vi "Render Inverted Section with Null.vi"(8 "Error In":errorcluster) -> (0 "Error Out":errorcluster)   [LabVIEW 2018, in "Tests.lvlib" / "Render.lvlib"]
uses:
  Render.lvlib
  <vilib>/addons/_JKI Toolkits/Caraya/classes/Test/Test.lvclass
  <vilib>/addons/_JKI Toolkits/Caraya/classes/Assert/Assert.lvclass
  src/Toolkit/Toolkit.lvlib
  src/Toolkit/Low-Level/Support/Render to String.vi
  src/Toolkit/Low-Level/Support/Lex String.vi
  src/Toolkit/Data/Null/Null.lvclass
  src/Toolkit/Low-Level/Context/Compiler.lvclass
  D:/Users/cfield/Code/Field R&D Services/Labstache/src/Toolkit/Data/Datum/Datum.lvclass
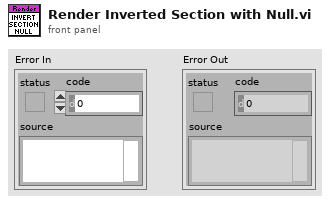
[diagram p1: front panel]
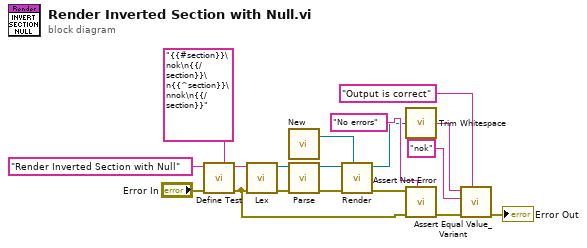
[diagram p0: block diagram]
diagram:
  n1 = call <vilib>:"Define Test.vi"("error in (no error)"="Error In", "Label (VI Title)"="Render Inverted Section with Null") -> ("error out"=w7:errorcluster)  [unwired: 9 in]
  n2 = call-poly "Lex.vi"("Error In"=w7, "Context In"="{{#section}}\nok\n{{/section}}\n{{^section}}\nnok\n{{/section}}" ("Input")) -> ("Error Out"=w8:errorcluster, "Context Out"=w9:refnum<class "Compiler.lvclass">)  [unwired: 7 in, 1 out]
  n3 = call "New.vi"() -> ("Null"=w1:refnum<class "Null.lvclass">)
  n4 = call "Parse.vi"("Error In"=w8, "Context In"=w9) -> ("Error Out"=w10:errorcluster, "Context Out"=w6:refnum<class "Compiler.lvclass">)  [unwired: 7 in, 1 out]
  n5 = call-poly "Render.vi"(7:w1, "Error In"=w10, "Context In"=w6) -> ("Error Out"=w11:errorcluster, "Context Out"=w3:refnum<class "Compiler.lvclass">)  [unwired: 6 in, 1 out]
  n6 = call <vilib>:"Trim Whitespace.vi"("string"=w3) -> ("trimmed string"=w2:string)  [unwired: 1 in]
  n7 = call <vilib>:"Assert Not Error.vi"("Label"="No errors", "error in (no error)"=w7, "Not Error?"=w11) -> ("error out"=w14:errorcluster)  [unwired: 8 in]
  n8 = call <vilib>:"Assert Equal Value_Variant.vi"("Label"="Output is correct", "error in (no error)"=w14, "Y"="nok", "X"=w2) -> ("error out"=→"Error Out":errorcluster)  [unwired: 7 in]
